vi "Check Debug Client Version.vi"(8 "error in (no error)":errorcluster, 10 "Debug Client Name":string) -> (0 "error out":errorcluster, 1 "DC Version":string, 2 "Valid":bool)   [LabVIEW 2017, in "DS TCP Server.lvlib" / "DS TCP Server.lvclass"]
uses:
  DS TCP Server.lvclass
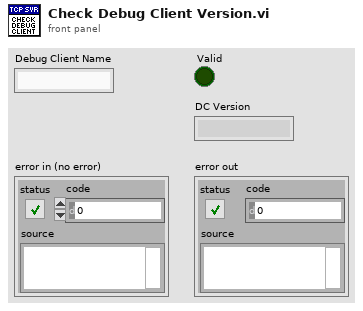
[diagram p1: front panel]
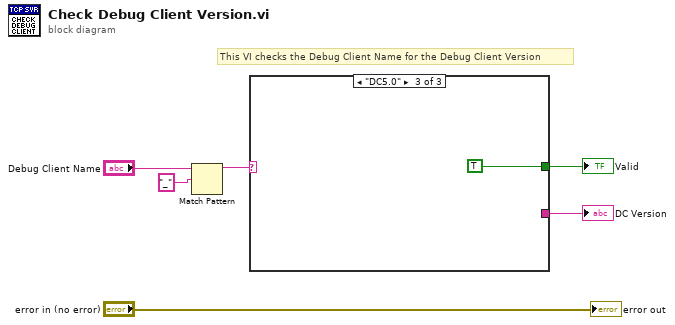
[diagram p0: block diagram]
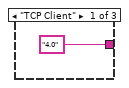
[diagram p2: hidden frame]
diagram:
  # "This VI checks the Debug Client Name for the Debug Client Version"
  n1 = Match Pattern(string="Debug Client Name", regular expression="_") -> (before substring=w3:string)  [unwired: 1 in, 3 out]
  n2 = case shown="\"DC5.0\"" w3 {
    selector: w3 -> [_ w8 _]
    tunnel: [_ _ TRUE] -> w2
    tunnel: ["4.0" w8 _] -> w1
    frame "TCP Client" {
    }
    frame Default {
    }
    frame "DC5.0" {
    }
  }
  "Valid" <- w2
  "DC Version" <- w1
  "error out" <- "error in (no error)"
